vi "Data FGV.vi"(7 "Operation":enum16{"Get", "Set"}(ring), 11 "DataMap":refnum<data-value>) -> (2 "DataMap Out":refnum<data-value>, 3 "Data":variant)   [LabVIEW 2017, in "Controller.lvlib" / "gController.lvclass"]
uses:
  gController.lvclass
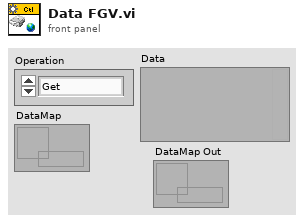
[diagram p1: front panel]
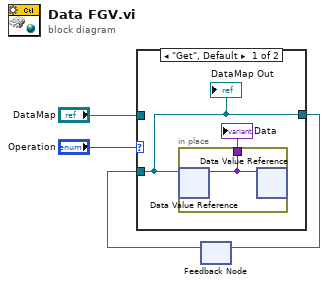
[diagram p0: block diagram]
diagram:
  n1 = feedback #1() -> (w1:refnum<data-value>)  [unwired: 1 in]
  n2 = case shown="\"Get\", Default" "Operation" {
    tunnel: "DataMap" -> [_ w8]
    tunnel: [w6 w8] -> w2
    tunnel: w1 -> [w6 _]
    frame "Get", Default {
      n3 = in-place {
        in-place-border: [w7] -> w5
        n4 = in-place-dvr #2(w6) -> (w7:variant)  [unwired: 1 out]
        n5 = in-place-dvr #2(w7) -> ()  [unwired: 2 out]
      }
      "Data" <- w5
      "DataMap Out" <- w6
    }
    frame "Set" {
    }
  }
  n6 = feedback-in #1(w2) -> ()
